vi "FindSymbolInDir.vi"(8 "error in (no error)":errorcluster, 11 "path":path) -> (0 "error out":errorcluster, 1 "String":string, 2 "Exits?":bool, 3 "path (dup)":path)   [LabVIEW 2013]
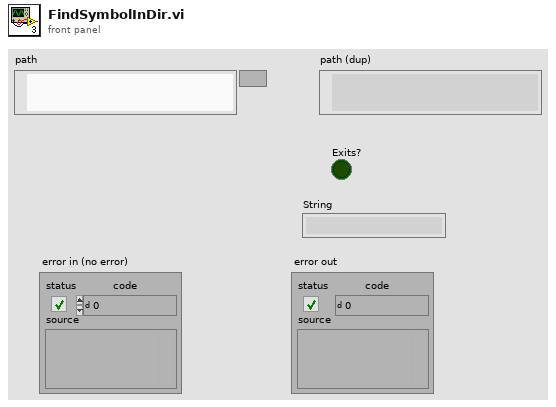
[diagram p1: front panel]
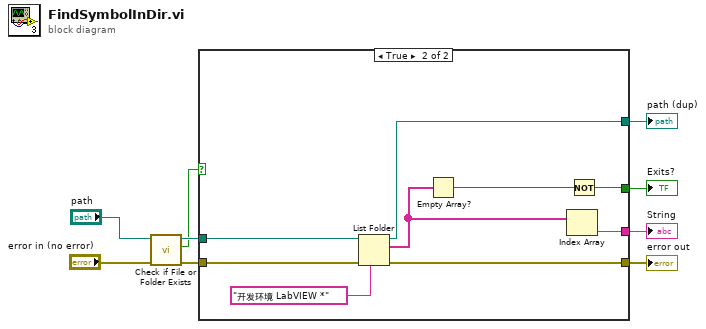
[diagram p0: block diagram]
diagram:
  n1 = call <vilib>:"Check if File or Folder Exists.vi"("error in (no error)"="error in (no error)", "path"="path") -> ("error out"=w6:errorcluster, "file or folder exists?"=w5:bool, "dup path"=w7:path)  [unwired: 7 in]
  n2 = case shown="True" w5 {
    tunnel: w7 -> [w10 w14]
    tunnel: w6 -> [w11 w20]
    tunnel: [w11 w19] -> w8
    tunnel: [_ w17] -> w3
    tunnel: [_ w16] -> w2
    tunnel: [w10 w15] -> w1
    frame False {
    }
    frame True {
      n3 = List Folder(path=w14, pattern="开发环境 LabVIEW *", error in=w20) -> (path out=w15:path, filenames=w12:string[], error out=w19:errorcluster)  [unwired: 1 in, 1 out]
      n4 = Empty Array?(array=w12) -> (empty?=w18:bool)
      n5 = Index Array(array=w12) -> (element=w16:string)  [unwired: 1 in]
      n6 = Not(x=w18) -> (.not. x?=w17:bool)
    }
  }
  "error out" <- w8
  "Exits?" <- w3
  "String" <- w2
  "path (dup)" <- w1
